vi "Get Decls.vi"(8 "error in (no error)":errorcluster, 11 "object in":refnum<class "SwitchCaseElement.lvclass">) -> (0 "error out":errorcluster, 2 "Declarations":refnum<class "CodeElement.lvclass">[](array[class]), 3 "object out":refnum<class "SwitchCaseElement.lvclass">)   [LabVIEW 2017, in "SwitchCaseElement.lvclass"]
uses:
  SwitchCaseElement.lvclass
  Base/CodeElement.lvclass
  SwitchCaseElement.lvclass/SwitchCaseElement.ctl
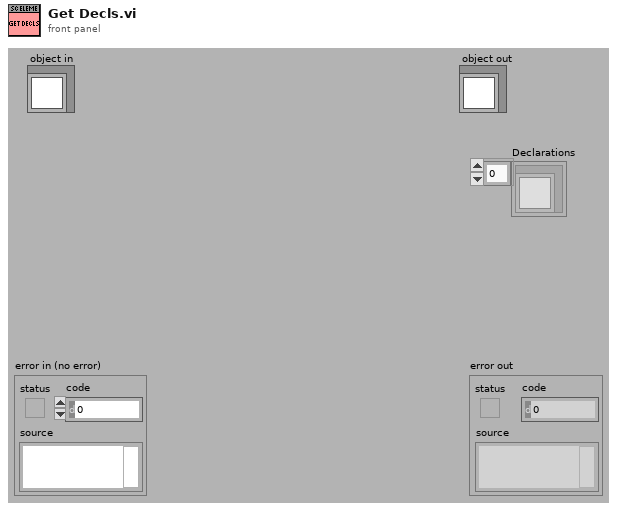
[diagram p1: front panel]
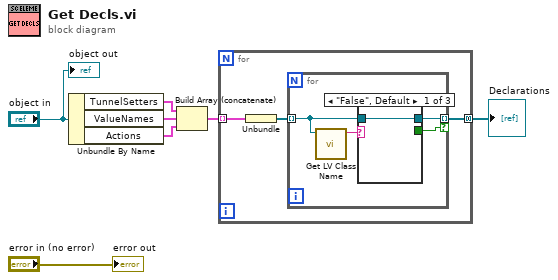
[diagram p0: block diagram]
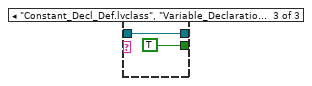
[diagram p3: hidden frame]
diagram:
  n1 = Unbundle By Name("object in") -> ("TunnelSetters"=w5:cluster{refnum<class "CodeElement.lvclass">[]}[], "ValueNames"=w4:cluster{refnum<class "CodeElement.lvclass">[]}[], "Actions"=w3:cluster{refnum<class "CodeElement.lvclass">[]}[])
  n2 = Build Array (concatenate)(w5, w4, w3) -> (w2:cluster{refnum<class "CodeElement.lvclass">[]}[])
  n3 = for {
    tunnel: w2 -> [w10] mode=indexing
    tunnel: [w8] -> w1 mode=concatenating
    n4 = Unbundle(w10) -> (w9:refnum<class "CodeElement.lvclass">[])
    n5 = for {
      tunnel: w9 -> [w13] mode=indexing
      tunnel: [w12] -> w8 mode=indexing if=w11
      n6 = call <vilib>:"Get LV Class Name.vi"("object"=w13) -> ("class name"=w14:string)  [unwired: 9 in, 1 out]
      n7 = case shown="\"False\", Default" w14 {
        tunnel: [w15 w16 w18] -> w12
        tunnel: w13 -> [w15 w16 w18]
        tunnel: [_ _ TRUE] -> w11
        frame "False", Default {
        }
        frame "SetInputValue.lvclass", "SetIntermediateValue.lvclass" {
        }
        frame "Constant_Decl_Def.lvclass", "Variable_Declaration.lvclass" {
        }
      }
    }
  }
  "Declarations" <- w1
  "error out" <- "error in (no error)"
  "object out" <- "object in"
